vi "Update Status.vi"(10 "Result":T1, 11 "Result Model in":refnum<class "Result Model.lvclass">) -> (3 "Result Model out":refnum<class "Result Model.lvclass">)   [LabVIEW 2020, in "Result Model.lvclass"]
uses:
  Result Model.lvclass
  Result Model.lvclass/Result Model.ctl
  <vilib>/Utility/miscctls.llb/LVMapReplaceAction.ctl
  Result/Status.ctl
  Result/Result.lvlib
  Result/Type.ctl
  Result/Result.ctl
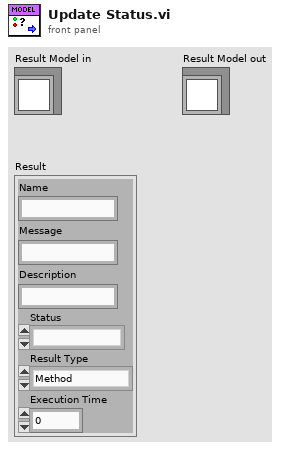
[diagram p1: front panel]
types:
  T1 = typedef "Result.lvlib/Result.ctl" = cluster{"Name":string, "Message":string, "Description":string, "Status":T2, "Result Type":T3, "Execution Time":dbl}
  T2 = typedef "Result.lvlib/Status.ctl" = enum16{"", "Passed", "Failed", "Error", "Skipped", "Setup Error", "Broken", "Teardown Error"}
  T3 = typedef "Result.lvlib/Type.ctl" = enum16{"Method", "Case", "Suite", "Pass", "Fail", "Skip", "Pass if", "Fail if", "Pass if Error", "Fail if Error", "Pass if Equal", "Fail if Equal"}
  T4 = typedef "LVMapReplaceAction.ctl" = enum32{"Modify Entry only if found", "Add or Modify Entry", "Delete Entry"}
  T5 = cluster{"Result Type":T3, "Status":T2, "Message":string, "Description":string}
  T6 = typedef "Result Model.lvclass/Model State.ctl" = cluster{"Run Queue":set{string}, "Test Statuses":map{string, T2}, "Execution Time":map{string, dbl}, "Assertions":map{string, cluster{"Result Type":T3, "Status":T2, "Message":string, "Description":string}[]}}
  T7 = map{string, cluster{"Result Type":T3, "Status":T2, "Message":string, "Description":string}[]}
  T8 = cluster{"Result Type":T3, "Status":T2, "Message":string, "Description":string}[]
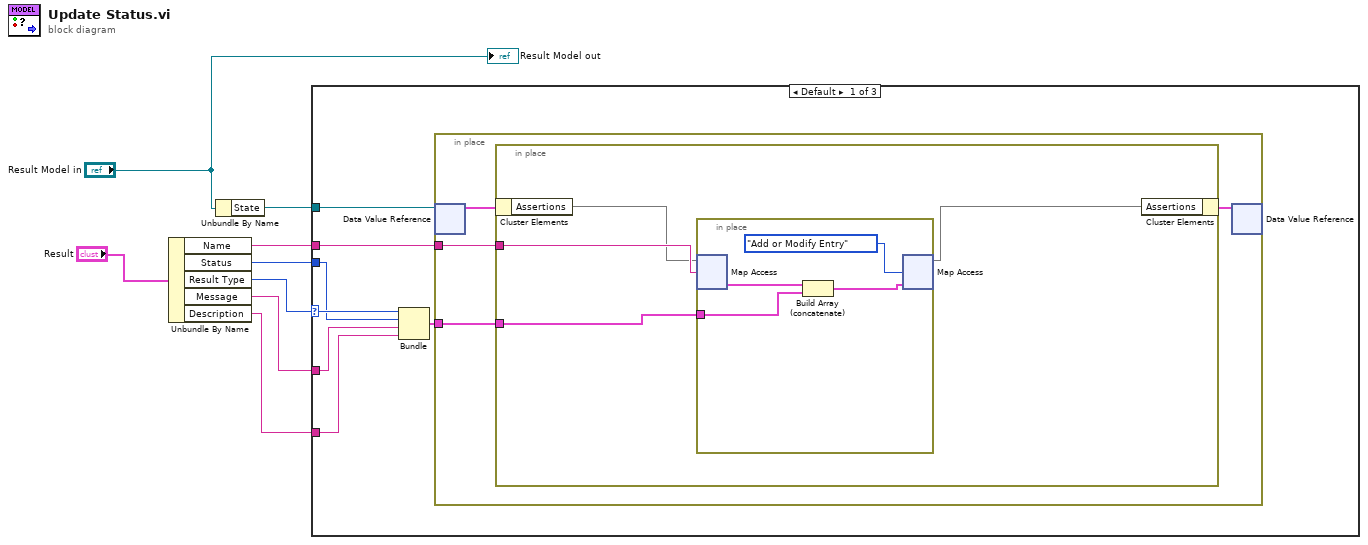
[diagram p0: block diagram]
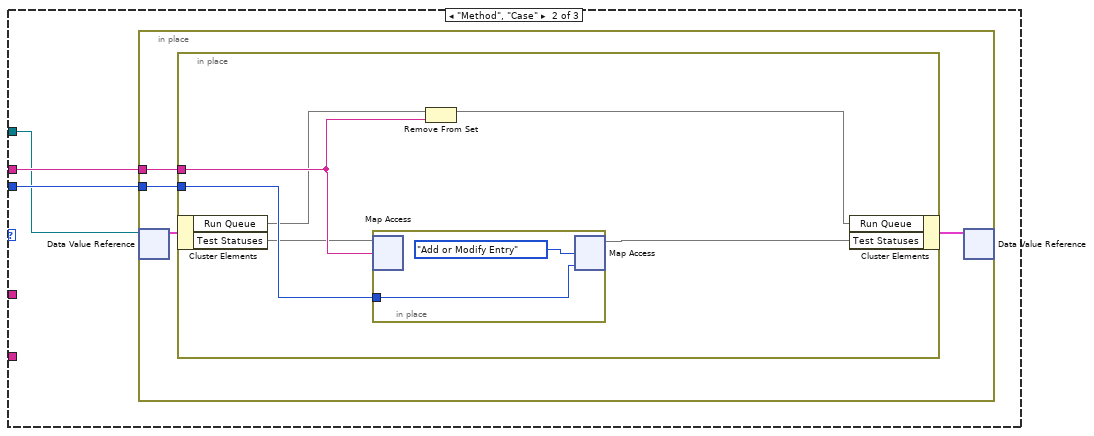
[diagram p2: hidden frame]
diagram:
  n1 = Unbundle By Name("Result") -> ("Name"=w8:string, "Status"=w7:T2, "Result Type"=w5:T3, "Message"=w4:string, "Description"=w3:string)
  n2 = Unbundle By Name("Result Model in") -> ("State"=w2:refnum<data-value>)
  n3 = case shown="Default" w5 {
    selector: w5 -> [w11 _ _]
    tunnel: w8 -> [w12 w30 _]
    tunnel: w7 -> [w10 w29 _]
    tunnel: w4 -> [w14 _ _]
    tunnel: w3 -> [w13 _ _]
    tunnel: w2 -> [w9 w28 _]
    frame Default {
      n4 = Bundle("Result Type"=w11, "Status"=w10, "Message"=w14, "Description"=w13) -> (w15:T5)  [unwired: 1 in]
      n5 = in-place {
        in-place-border: w15 -> [w19]
        in-place-border: w12 -> [w18]
        n6 = in-place-dvr #1(w9) -> (w17:T6)  [unwired: 1 out]
        n7 = in-place {
          in-place-border: w19 -> [w23]
          in-place-border: w18 -> [w22]
          n8 = in-place-cluster #2(w17) -> ("Assertions"=w21:T7)
          n9 = in-place {
            in-place-border: w23 -> [w25]
            n10 = in-place-map #3(w21, w22) -> (w27:T8)  [unwired: 1 in, 1 out]
            n11 = Build Array (concatenate)(w27, w25) -> (w26:T8)
            n12 = in-place-map #3(w26, LVMapReplaceAction."Add or Modify Entry" ("action")) -> (w20:T7)  [unwired: 2 out]
          }
          n13 = in-place-cluster #2("Assertions"=w20) -> (w16:T6)
        }
        n14 = in-place-dvr #1(w16) -> ()  [unwired: 2 out]
      }
    }
    frame "Method", "Case" {
      n15 = in-place {
        in-place-border: w30 -> [w34]
        in-place-border: w29 -> [w33]
        n16 = in-place-dvr #4(w28) -> (w32:T6)  [unwired: 1 out]
        n17 = in-place {
          in-place-border: w34 -> [w40]
          in-place-border: w33 -> [w39]
          n18 = in-place-cluster #5(w32) -> ("Run Queue"=w38:set{string}, "Test Statuses"=w37:map{string, T2})
          n19 = in-place {
            in-place-border: w39 -> [w41]
            n20 = in-place-map #6(w37, w40) -> ()  [unwired: 1 in, 2 out]
            n21 = in-place-map #6(w41, LVMapReplaceAction."Add or Modify Entry" ("action")) -> (w35:map{string, T2})  [unwired: 2 out]
          }
          n22 = Remove From Set(10:w40, 11:w38) -> (3:w36:set{string})  [unwired: 1 out]
          n23 = in-place-cluster #5("Run Queue"=w36, "Test Statuses"=w35) -> (w31:T6)
        }
        n24 = in-place-dvr #4(w31) -> ()  [unwired: 2 out]
      }
    }
    frame "Suite" {
    }
  }
  "Result Model out" <- "Result Model in"
